vi "ref_rotary_PKP214_masterslave.vi"() -> ()   [LabVIEW 2014]
uses:
  <vilib>/eio/EIONode/EIONode.xnode
  <vilib>/rvi/FXPMathLib/FxpMul/XNode/nifxpmath_Multiplier.xnode
  <vilib>/rvi/FXPMathLib/sim/FxpSim.dll
  <vilib>/rvi/eio/common/nirviEmuTemplateMethod_errors.vi
  <vilib>/rvi/FXPMathLib/FxpSinAndCos/XNode/nifxpmath_SinAndCos.xnode
  <vilib>/rvi/FXPMathLib/FxpSinAndCos/simVIs/DllFxpSinAndCosTemp_sub.vi
  <vilib>/rvi/FXPMathLib/FxpSinAndCos/subVIs/nifxpmath_SinAndCos_SimConfig.ctl
  <vilib>/rvi/FXPMathLib/FxpSub/XNode/nifxpmath_Sub.xnode
  <vilib>/rvi/FXPMathLib/FxpAdd/XNode/nifxpmath_Add.xnode
  <vilib>/rvi/DataTransferAndStorage/Container/XNode/niFpgaContainer.xnode
  <vilib>/rvi/interface/RandomDataEmulation/nirviRandomDataFpgaMultiElementTemplate.vi
panel:
  out "omega_a (M_avg) 2":fxp<+/-,64,35>
  in  "Velocity Estimation":i16(ring) items=["M_avg method", "T method"]
  out "omega_a (M_avg)":fxp<+/-,64,35>
  in  "D_d_M_avg_Tc (uSec)":u32
  in  "theta_a_tolorence":fxp<+/-,14,3>
  in  "theta2 ratio":fxp<+/-,20,8>
  in  "tauk ratio":fxp<+/-,20,8>
  in  "tauk2_tol":fxp<+/-,20,8>
  in  "masterslave":bool
  out "Theta_ar 2":fxp<+/-,54,19>
  in  "stop motor 2":bool
  out "vb 2":fxp<+/-,38,8>
  out "va 2":fxp<+/-,38,8>
  out "vd_F 2":fxp<+/-,20,5>
  out "vq_F 2":fxp<+/-,20,5> format="%.57g"
  out "taukr_dd 2":fxp<+/-,36,29>
  out "tauk_i 2":fxp<+/-,34,18>
  in  "Kv 2":fxp<+/-,20,12>
  in  "Bv 2":fxp<+/-,20,2>
  out "taukr 2":fxp<+/-,64,31>
  out "Theta_a_error 2":fxp<+/-,24,11>
  in  "Kp 2":fxp<+/-,20,12>
  in  "Kd 2":fxp<+/-,20,8>
  out "taur 2":fxp<+/-,64,31>
  out "tauk_error 2":fxp<+/-,24,11>
  in  "Ki 2":fxp<+/-,22,9>
  in  "tauk_tolorence 2":fxp<+/-,14,3>
  out "tauk_dd 2":fxp<+/-,34,18>
  out "tauk 2":fxp<+/-,34,13>
  in  "Reduction ratio 2":fxp<+/-,20,6>
  in  "Spring stiffness 2":fxp<+/-,20,12>
  out "omega_a (rad/s)  2":fxp<+/-,32,18>
  out "omega (rad/s) 2":fxp<+/-,32,18>
  out "omega_a(T) 2":fxp<+/-,20,9>
  in  "Magnetic Encoder Reset 2":bool
  out "Magnetic Encoder Position 2":i32
  out "Theta_a 2":fxp<+/-,34,12>
  in  "Correction factor 2":fxp<+/-,24,2>
  out "mt 2":u32
  out "omega(T) 2":fxp<+/-,20,9>
  in  "Encoder Reset 2":bool
  out "Encoder Position 2":i32
  out "NrTheta 2":fxp<+/-,33,18>
  out "Thetam 2":fxp<+/-,33,18>
  in  "Correction factor":fxp<+/-,24,2>
  in  "Reduction ratio":fxp<+/-,20,6>
  out "tauk_dd":fxp<+/-,34,18>
  out "tauk":fxp<+/-,34,12>
  in  "Spring stiffness":fxp<+/-,20,12>
  in  "Kp":fxp<+/-,20,12>
  in  "Kd":fxp<+/-,20,8>
  out "taur":fxp<+/-,64,31>
  out "tauk_error":fxp<+/-,24,11>
  in  "Ki":fxp<+/-,22,9>
  in  "tauk_tolorence":fxp<+/-,14,3>
  out "omega_a (rad/s)":fxp<+/-,32,18>
  out "omega_a(T)":fxp<+/-,32,15>
  out "Theta_ar_dd":fxp<+/-,36,29>
  in  "Magnetic Encoder Reset":bool
  out "Magnetic Encoder Position":i32
  out "Theta_a":fxp<+/-,34,11>
  out "Thetam":fxp<+/-,33,18>
  out "omega(T)":fxp<+/-,32,15>
  out "Time now (s)":fxp<+,52,14>
  out "Theta_ar":fxp<+,1,1>
  out "tauk_i":fxp<+/-,34,18>
  out "Theta_a_error":fxp<+/-,24,11>
  out "taukr":fxp<+/-,64,31>
  in  "Bv":fxp<+/-,20,8>
  in  "Kv":fxp<+/-,20,12>
  out "taukr_dd":fxp<+/-,36,29>
  in  "Ini coe.":bool
  out "va":fxp<+/-,38,8>
  out "vb":fxp<+/-,38,8>
  in  "stop motor":bool
  out "vq_F":fxp<+/-,20,5> format="%.57g"
  out "vd_F":fxp<+/-,20,5>
  out "mt":u32
  out "omega (rad/s)":fxp<+/-,32,18>
  in  "mt0":u32
  out "NrTheta":fxp<+/-,33,18>
  out "Encoder Position":i32
  in  "Encoder Reset":bool
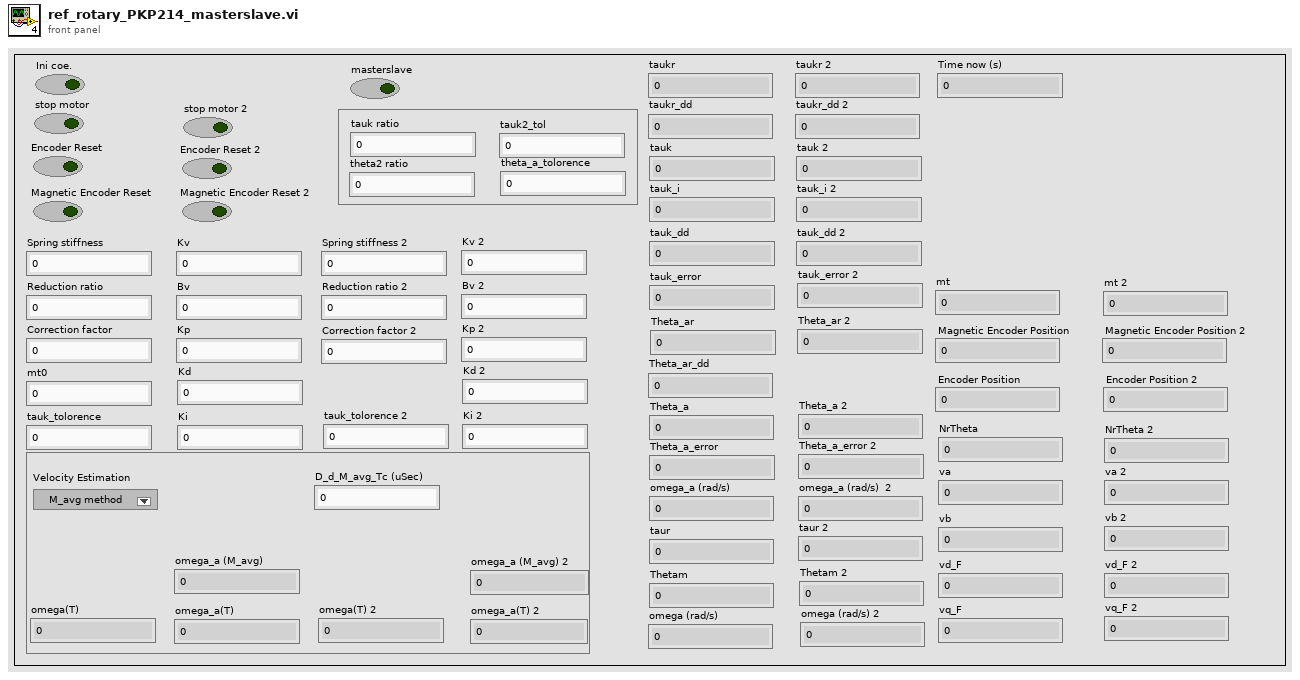
[diagram p1: front panel]
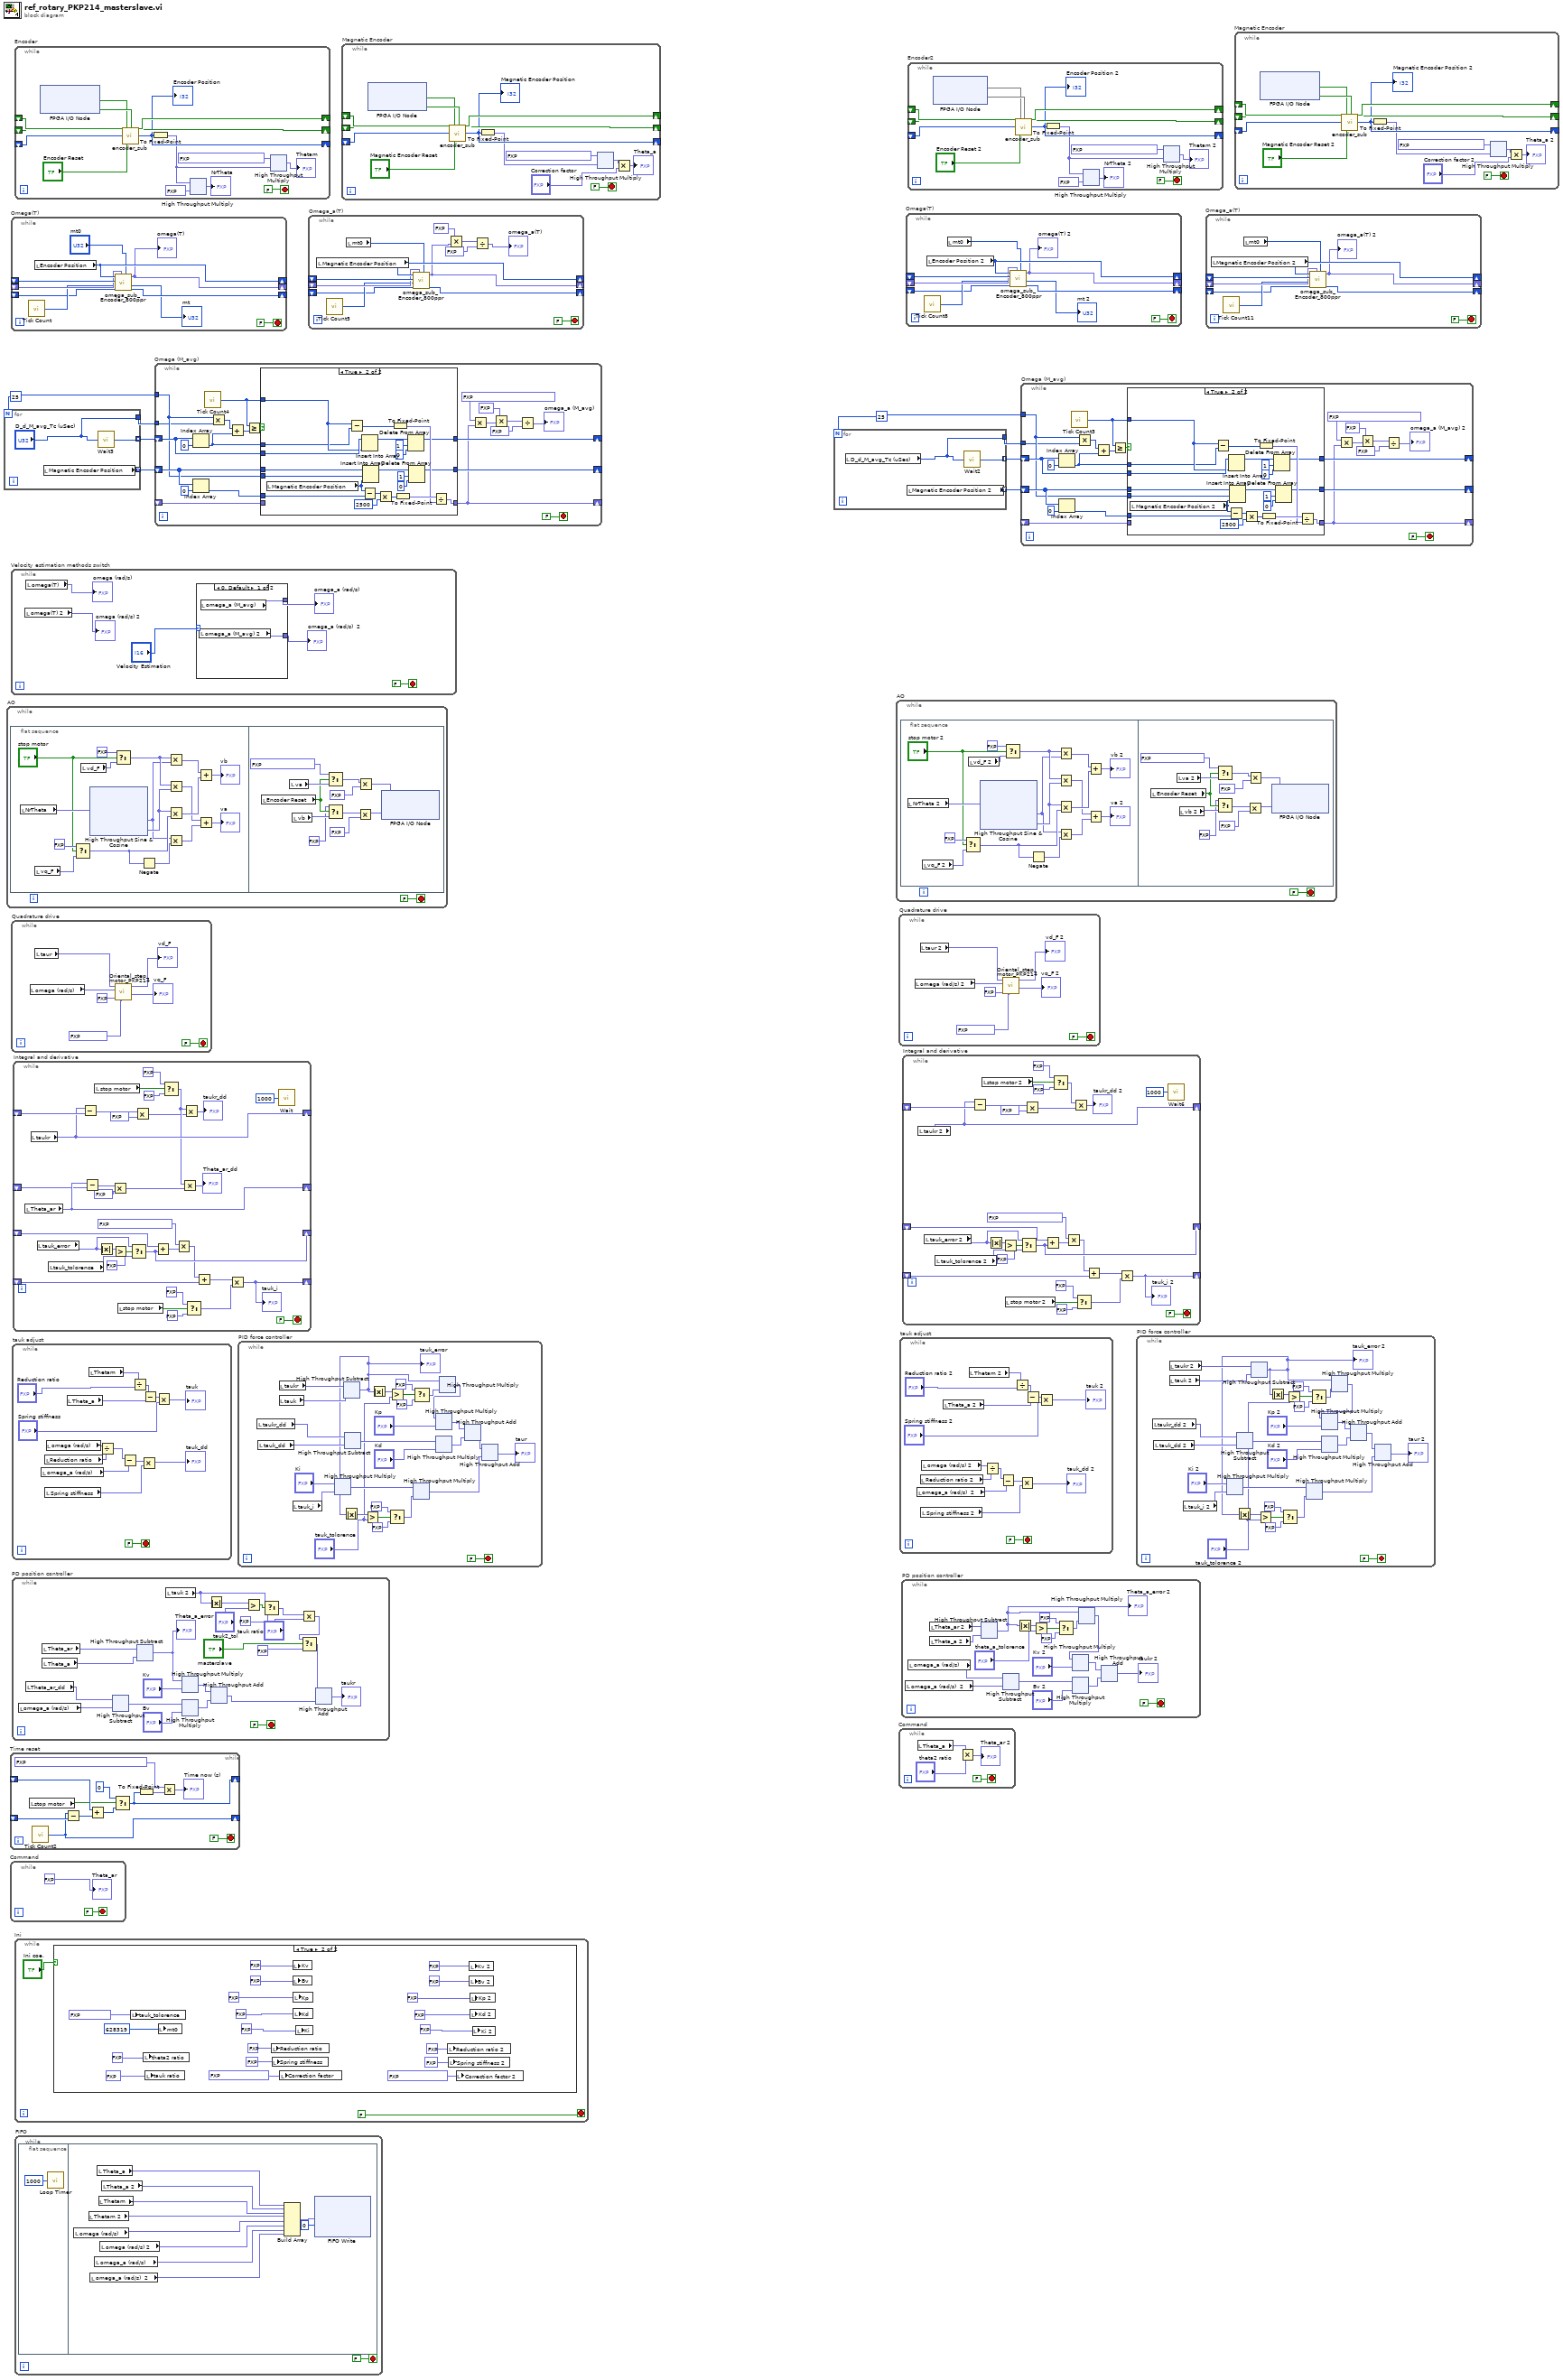
[diagram p0: block diagram]
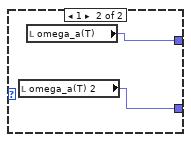
[diagram p4: hidden frame]
diagram:
  w1 = 25
  w5 = 25
  n1 = for {
    N: w5 -> [_]
    tunnel: ["D_d_M_avg_Tc (uSec)"] -> w8
    tunnel: [w11] -> w6 mode=indexing
    tunnel: [w10] -> w7 mode=indexing
    n2 = local read "Magnetic Encoder Position"() -> (w10:i32)
    n3 = call "Wait3"("Count(uSec)"="D_d_M_avg_Tc (uSec)") -> ("Tick Count(uSec)"=w11:u32)
  }
  n4 = while "AO" {
    stop <- FALSE stop-if-true
    n5 = flat-sequence {
      frame #0 {
        n6 = local read "NrTheta"() -> (w28:fxp<+/-,33,18>)
        n7 = local read "vq_F"() -> (w26:fxp<+/-,20,5>)
        n8 = Select(t=fxp<+,20,5> 0.0, s="stop motor", f=w26) -> (s? t:f=w23:fxp<+/-,21,6>)
        n9 = local read "vd_F"() -> (w27:fxp<+/-,20,5>)
        n10 = xnode "High Throughput Sine & Cosine"("x (pi)"=w28) -> ("sin(x)"=w19:fxp<+/-,17,2>, "cos(x)"=w21:fxp<+/-,17,2>)
        n11 = Select(t=fxp<+,20,5> 0.0, s="stop motor", f=w27) -> (s? t:f=w20:fxp<+/-,21,6>)
        n12 = Negate(x=w23) -> (-x=w22:fxp<+/-,21,6>)
        n13 = Multiply(x=w20, y=w19) -> (x*y=w18:fxp<+/-,37,7>)
        n14 = Multiply(x=w20, y=w21) -> (x*y=w16:fxp<+/-,37,7>)
        n15 = Multiply(x=w21, y=w23) -> (x*y=w17:fxp<+/-,37,7>)
        n16 = Multiply(x=w19, y=w22) -> (x*y=w15:fxp<+/-,37,7>)
        n17 = Add(x=w18, y=w17) -> (x+y=→"vb":fxp<+/-,38,8>)
        n18 = Add(x=w16, y=w15) -> (x+y=→"va":fxp<+/-,38,8>)
      }
      frame #1 {
        n19 = local read "Encoder Reset"() -> (w62:bool)
        n20 = local read "va"() -> (w64:fxp<+/-,38,8>)
        n21 = local read "vb"() -> (w63:fxp<+/-,38,8>)
        n22 = Select(t=fxp<+/-,20,5> 3.899993896484375 ("y"), s=w62, f=w64) -> (s? t:f=w65:fxp<+/-,38,8>)
        n23 = Select(t=fxp<+/-,20,5> 0.0 ("y"), s=w62, f=w63) -> (s? t:f=w66:fxp<+/-,38,8>)
        n24 = Multiply(x=w66, y=fxp<+/-,20,5> -0.5) -> (x*y=w70:fxp<+/-,57,12>)
        n25 = Multiply(x=w65, y=fxp<+/-,20,5> -0.5) -> (x*y=w69:fxp<+/-,57,12>)
        n26 = xnode "FPGA I/O Node"("Mod2/AO0"=w69, "Mod2/AO1"=w70) -> ()  [unwired: 2 in, 2 out]
      }
    }
  }
  n27 = while "Time reset" {
    shift-right: [w74] -> _
    shift-left: _ -> [w81]
    shift-right: [w76] -> _
    shift-left: _ -> [w77]
    stop <- FALSE stop-if-true
    n28 = local read "stop motor"() -> (w79:bool)
    n29 = call "Tick Count2"() -> ("Tick Count(uSec)"=w76:u32)
    n30 = Subtract(x=w76, y=w77) -> (x-y=w82:u32)
    n31 = Add(x=w81, y=w82) -> (x+y=w80:u32)
    n32 = Select(t=u32 0, s=w79, f=w80) -> (s? t:f=w74:u32)
    n33 = To Fixed-Point(number=w74) -> (fixed-point=w73:fxp<+,32,32>)  [unwired: 1 in]
    n34 = Multiply(x=fxp<+,20,-18> 1.0000003385357559e-06, y=w73) -> (x*y=→"Time now (s)":fxp<+,52,14>)
  }
  n35 = while "Command" {
    stop <- FALSE stop-if-true
    "Theta_ar" <- fxp<+,1,1> 0.0 ("t")
  }
  n36 = while "Omega(T)" {
    shift-right: [w93] -> _
    shift-left: _ -> [w94]
    shift-right: [w85] -> _
    shift-left: _ -> [w92]
    shift-right: [w89] -> _
    shift-left: _ -> [w90]
    stop <- FALSE stop-if-true
    n37 = call "Tick Count"() -> ("Tick Count(Ticks)"=w91:u32)
    n38 = local read "Encoder Position"() -> (w93:i32)
    n39 = call "omega_sub_Encoder_800ppr.vi"("mt0"="mt0", "omega_pre"=w92, "ticks_m_pre"=w90, "ticks"=w91, "count_pre"=w94, "count"=w93) -> ("ticks_m"=w89:u32, "mt"=→"mt":u32, "omega"=w85:fxp<+/-,20,9>)  [unwired: 3 in]
    "omega(T)" <- w85
  }
  n40 = while "Velocity estimation methods switch" {
    stop <- FALSE stop-if-true
    n41 = local read "omega(T) 2"() -> (→"omega (rad/s) 2":fxp<+/-,20,9>)
    n42 = local read "omega(T)"() -> (→"omega (rad/s)":fxp<+/-,32,15>)
    n43 = case shown="0, Default" "Velocity Estimation" {
      tunnel: [w102 w104] -> w97
      tunnel: [w101 w103] -> w96
      frame 0, Default {
        n44 = local read "omega_a (M_avg) 2"() -> (w101:fxp<+/-,64,35>)
        n45 = local read "omega_a (M_avg)"() -> (w102:fxp<+/-,64,35>)
      }
      frame 1 {
        n46 = local read "omega_a(T) 2"() -> (w103:fxp<+/-,20,9>)
        n47 = local read "omega_a(T)"() -> (w104:fxp<+/-,32,15>)
      }
    }
    "omega_a (rad/s)" <- w97
    "omega_a (rad/s)  2" <- w96
  }
  n48 = while "Quadrature drive" {
    stop <- FALSE stop-if-true
    n49 = local read "omega (rad/s)"() -> (w109:fxp<+/-,32,18>)
    n50 = local read "taur"() -> (w110:fxp<+/-,64,31>)
    n51 = call "Oriental_step_motor_PKP214.vi"("tau_Threshold"=fxp<+,16,7> 0.00390625 ("F_Threshold"), "dtaumr"=fxp<+/-,25,15> 0.0 ("dFmr"), "omega"=w109, "taumr"=w110) -> ("vq_F"=→"vq_F":fxp<+/-,20,5>, "vd_F"=→"vd_F":fxp<+/-,20,5>)  [unwired: 6 in]
  }
  n52 = while "PD position controller" {
    stop <- FALSE stop-if-true
    n53 = local read "omega_a (rad/s)"() -> (w126:fxp<+/-,32,18>)
    n54 = local read "Theta_ar_dd"() -> (w125:fxp<+/-,36,29>)
    n55 = local read "Theta_ar"() -> (w128:fxp<+,1,1>)
    n56 = local read "Theta_a"() -> (w135:fxp<+/-,34,11>)
    n57 = xnode "High Throughput Subtract"("x"=w125, "y"=w126) -> ("x-y"=w127:fxp<+/-,44,30>)
    n58 = xnode "High Throughput Subtract"("x"=w128, "y"=w135) -> ("x-y"=w129:fxp<+/-,35,12>)
    "Theta_a_error" <- w129
    n59 = local read "tauk 2"() -> (w119:fxp<+/-,34,13>)
    n60 = xnode ("High Throughput Multiply")("x"=w129, "y"="Kv") -> ("x*y"=w133:fxp<+/-,55,24>)
    n61 = xnode ("High Throughput Multiply")("x"=w127, "y"="Bv") -> ("x*y"=w132:fxp<+/-,64,38>)
    n62 = Absolute Value(x=w119) -> (abs(x)=w117:fxp<+,34,13>)
    n63 = xnode ("High Throughput Add")("x"=w133, "y"=w132) -> ("x+y"=w124:fxp<+/-,64,39>)
    n64 = Greater?(x=w117, y="tauk2_tol") -> (0:w118:bool)
    n65 = Select(t=w119, s=w118, f=fxp<+,1,1> 0.0 ("t")) -> (s? t:f=w113:fxp<+/-,34,13>)
    n66 = Multiply(x=w113, y="tauk ratio") -> (x*y=w114:fxp<+/-,54,21>)
    n67 = Select(t=w114, s="masterslave", f=fxp<+,1,1> 0.0 ("t")) -> (s? t:f=w120:fxp<+/-,54,21>)
    n68 = xnode ("High Throughput Add")("x"=w120, "y"=w124) -> ("x+y"=→"taukr":fxp<+/-,64,40>)
  }
  n69 = while "tauk adjust" {
    stop <- FALSE stop-if-true
    n70 = local read "omega_a (rad/s)"() -> (w147:fxp<+/-,32,18>)
    n71 = local read "Reduction ratio"() -> (w144:fxp<+/-,20,6>)
    n72 = local read "Spring stiffness"() -> (w145:fxp<+/-,20,12>)
    n73 = local read "omega (rad/s)"() -> (w146:fxp<+/-,32,18>)
    n74 = local read "Theta_a"() -> (w141:fxp<+/-,34,11>)
    n75 = local read "Thetam"() -> (w140:fxp<+/-,33,18>)
    n76 = Divide(x=w146, y=w144) -> (x/y=w148:fxp<+/-,53,33>)
    n77 = Subtract(x=w148, y=w147) -> (x-y=w149:fxp<+/-,53,33>)
    n78 = Divide(x=w140, y="Reduction ratio") -> (x/y=w142:fxp<+/-,54,33>)
    n79 = Multiply(x=w149, y=w145) -> (x*y=→"tauk_dd":fxp<+/-,64,44>)
    n80 = Subtract(x=w142, y=w141) -> (x-y=w143:fxp<+/-,56,33>)
    n81 = Multiply(x=w143, y="Spring stiffness") -> (x*y=→"tauk":fxp<+/-,64,44>)
  }
  n82 = while "Integral and derivative" {
    shift-right: [w181] -> _
    shift-left: _ -> [w184]
    shift-right: [w173] -> _
    shift-left: _ -> [w174]
    shift-right: [w163] -> _
    shift-left: _ -> [w167]
    shift-right: [w160] -> _
    shift-left: _ -> [w159]
    stop <- FALSE stop-if-true
    n83 = local read "Theta_ar"() -> (w160:fxp<+,1,1>)
    n84 = local read "taukr"() -> (w181:fxp<+/-,64,31>)
    n85 = local read "tauk_error"() -> (w175:fxp<+/-,24,11>)
    n86 = local read "tauk_tolorence"() -> (w178:fxp<+/-,14,3>)
    n87 = Subtract(x=w181, y=w184) -> (x-y=w183:fxp<+/-,64,32>)
    n88 = Subtract(x=w160, y=w159) -> (x-y=w162:fxp<+,1,1>)
    n89 = local read "stop motor"() -> (w156:bool)
    n90 = Absolute Value(x=w175) -> (abs(x)=w179:fxp<+,24,11>)
    n91 = Multiply(x=w162, y=fxp<+/-,33,13> 1000.0) -> (x*y=w153:fxp<+,1,-19>)
    n92 = Greater?(x=w179, y=w178) -> (0:w177:bool)
    n93 = local read "stop motor"() -> (w170:bool)
    n94 = Select(t=w175, s=w177, f=fxp<+,24,11> 0.0) -> (s? t:f=w173:fxp<+/-,25,12>)
    n95 = Multiply(x=w183, y=fxp<+/-,33,13> 1000.0) -> (x*y=w151:fxp<+/-,64,44>)
    n96 = Add(x=w174, y=w173) -> (x+y=w172:fxp<+/-,26,13>)
    n97 = Select(t=fxp<+,1,1> 0.0, s=w156, f=fxp<+,1,1> 1.0) -> (s? t:f=w152:fxp<+,1,1>)
    n98 = Multiply(x=fxp<+/-,30,12> 0.000499725341796875, y=w172) -> (x*y=w166:fxp<+/-,55,24>)
    n99 = Multiply(x=w152, y=w153) -> (x*y=→"Theta_ar_dd":fxp<+,1,-19>)
    n100 = Multiply(x=w152, y=w151) -> (x*y=→"taukr_dd":fxp<+/-,64,44>)
    n101 = Select(t=fxp<+,1,1> 0.0, s=w170, f=fxp<+,1,1> 1.0) -> (s? t:f=w164:fxp<+,1,1>)
    n102 = Add(x=w166, y=w167) -> (x+y=w165:fxp<+/-,32,16>)
    n103 = Multiply(x=w165, y=w164) -> (x*y=w163:fxp<+/-,32,16>)
    "tauk_i" <- w163
    n104 = call "Wait"("Count(uSec)"=u32 1000) -> ()  [unwired: 1 out]
  }
  n105 = while "Encoder" {
    shift-right: [w194] -> _
    shift-left: _ -> [w196]
    shift-right: [w193] -> _
    shift-left: _ -> [w195]
    shift-right: [w191] -> _
    shift-left: _ -> [w192]
    stop <- FALSE stop-if-true
    n106 = xnode "FPGA I/O Node"() -> ("Mod7/DIO2"=w199:bool, "Mod7/DIO3"=w200:bool)  [unwired: 2 in, 2 out]
    n107 = call "encoder_sub.vi"("A_pre"=w196, "B_pre"=w195, "Encoder Position_pre"=w192, "A input"=w199, "Encoder Position Reset"="Encoder Reset", "B input"=w200) -> ("A"=w194:bool, "B"=w193:bool, "Encoder Position (Counts)"=w191:i32)  [unwired: 19 in]
    "Encoder Position" <- w191
    n108 = To Fixed-Point(number=w191) -> (fixed-point=w187:fxp<+/-,32,32>)  [unwired: 1 in]
    n109 = xnode ("High Throughput Multiply")("x"=w187, "y"=fxp<+/-,24,0> 0.125) -> ("x*y"=→"NrTheta":fxp<+/-,56,32>)
    n110 = xnode ("High Throughput Multiply")("x"=fxp<+/-,24,0> 0.007853984832763672 ("y"), "y"=w187) -> ("x*y"=→"Thetam":fxp<+/-,56,32>)
  }
  n111 = while "Ini" {
    stop <- FALSE stop-if-true
    n112 = case shown="True" "Ini coe." {
      frame False {
      }
      frame True {
        n113 = local write "tauk_tolorence"(fxp<+/-,14,3> 0.009765625 ("D_tolorence")) -> ()
        n114 = local write "theta2 ratio"(fxp<+/-,16,2> 1.0 ("Dr_end")) -> ()
        n115 = local write "tauk ratio"(fxp<+/-,16,2> -0.5 ("Dr_end")) -> ()
        n116 = local write "mt0"(u32 628319 ("mt0")) -> ()
        n117 = local write "Reduction ratio"(fxp<+/-,16,11> 18.0 ("Dr_end")) -> ()
        n118 = local write "Spring stiffness"(fxp<+/-,16,11> 1.5 ("Dr_end")) -> ()
        n119 = local write "Correction factor"(fxp<+/-,16,2> 0.97235107421875 ("Dr_end")) -> ()
        n120 = local write "Kv"(fxp<+/-,16,11> 0.0 ("Dr_end")) -> ()
        n121 = local write "Bv"(fxp<+/-,16,11> 0.0 ("Dr_end")) -> ()
        n122 = local write "Kp"(fxp<+/-,20,12> 1.0 ("Kp")) -> ()
        n123 = local write "Kd"(fxp<+/-,20,8> 0.0 ("Kd")) -> ()
        n124 = local write "Ki"(fxp<+/-,24,8> 0.0 ("D_i")) -> ()
        n125 = local write "Reduction ratio 2"(fxp<+/-,16,11> 18.0 ("Dr_end")) -> ()
        n126 = local write "Spring stiffness 2"(fxp<+/-,16,11> 1.5 ("Dr_end")) -> ()
        n127 = local write "Correction factor 2"(fxp<+/-,16,2> 0.97235107421875 ("Dr_end")) -> ()
        n128 = local write "Kv 2"(fxp<+/-,16,11> 1.0 ("Dr_end")) -> ()
        n129 = local write "Bv 2"(fxp<+/-,16,11> 0.0 ("Dr_end")) -> ()
        n130 = local write "Kp 2"(fxp<+/-,20,12> 1.0 ("Kp")) -> ()
        n131 = local write "Kd 2"(fxp<+/-,20,8> 0.0 ("Kd")) -> ()
        n132 = local write "Ki 2"(fxp<+/-,24,8> 0.0 ("D_i")) -> ()
      }
    }
  }
  n133 = while "FIFO" {
    stop <- FALSE stop-if-true
    n134 = flat-sequence {
      frame #0 {
        n135 = call "Loop Timer"("Count(uSec)"=u32 1000) -> ()  [unwired: 1 out]
      }
      frame #1 {
        n136 = local read "omega (rad/s)"() -> (w225:fxp<+/-,32,18>)
        n137 = local read "Thetam 2"() -> (w229:fxp<+/-,33,18>)
        n138 = local read "omega_a (rad/s)  2"() -> (w226:fxp<+/-,32,18>)
        n139 = local read "omega_a (rad/s)"() -> (w227:fxp<+/-,32,18>)
        n140 = local read "Theta_a"() -> (w232:fxp<+/-,34,11>)
        n141 = local read "Thetam"() -> (w230:fxp<+/-,33,18>)
        n142 = local read "omega (rad/s) 2"() -> (w228:fxp<+/-,32,18>)
        n143 = local read "Theta_a 2"() -> (w231:fxp<+/-,34,12>)
        n144 = Build Array(w232, w231, w230, w229, w225, w228, w227, w226) -> (w233:fxp<+/-,41,18>[])
        n145 = xnode ("FIFO Write")("Element"=w233, "Timeout"=0) -> ()  [unwired: 1 in, 2 out]
      }
    }
  }
  n146 = while "Omega (M_avg)" {
    tunnel: w5 -> [w250]
    shift-right: [w243] -> _
    shift-left: w6 -> [w254]
    shift-right: [w242] -> _
    shift-left: _ -> [w245]
    shift-right: [w244] -> _
    shift-left: w7 -> [w253]
    tunnel: w8 -> [w247]
    stop <- FALSE stop-if-true
    n147 = Index Array(array=w254, index=0) -> (element=w248:u32)
    n148 = Index Array(array=w253, index=0) -> (element=w249:i32)
    n149 = call "Tick Count4"() -> ("Tick Count(uSec)"=w251:u32)
    n150 = Multiply(x=w250, y=w247) -> (x*y=w255:u32)
    n151 = Add(x=w255, y=w248) -> (x+y=w252:u32)
    n152 = Greater Or Equal?(x=w251, y=w252) -> (x >= y?=w246:bool)
    n153 = case shown="True" w246 {
      tunnel: w254 -> [w260 w277]
      tunnel: w253 -> [w259 w276]
      tunnel: w251 -> [_ w269]
      tunnel: w250 -> [_ w275]
      tunnel: w249 -> [_ w273]
      tunnel: w248 -> [_ w268]
      tunnel: w245 -> [w258 _]
      tunnel: [w259 w263] -> w244
      tunnel: [w260 w262] -> w243
      tunnel: [w258 w261] -> w242
      frame False {
      }
      frame True {
        n154 = local read "Magnetic Encoder Position"() -> (w274:i32)
        n155 = Subtract(x=w269, y=w268) -> (x-y=w266:u32)
        n156 = Insert Into Array(array=w277, new element=w269) -> (w278:u32[])  [unwired: 1 in]
        n157 = Subtract(x=w274, y=w273) -> (x-y=w272:i32)
        n158 = Insert Into Array(array=w276, index=w275, new element=w274) -> (w279:i32[])
        n159 = Multiply(x=w272, y=2500) -> (x*y=w270:i32)
        n160 = To Fixed-Point(number=w266) -> (fixed-point=w264:fxp<+,32,32>)  [unwired: 1 in]
        n161 = To Fixed-Point(number=w270) -> (fixed-point=w265:fxp<+/-,32,32>)  [unwired: 1 in]
        n162 = Delete From Array(array=w278, length=1, index=0) -> (array with subset deleted=w262:u32[])  [unwired: 1 out]
        n163 = Delete From Array(array=w279, length=1, index=0) -> (array with subset deleted=w263:i32[])  [unwired: 1 out]
        n164 = Divide(x=w265, y=w264) -> (x/y=w261:fxp<+/-,64,32>)
      }
    }
    n165 = Multiply(x=fxp<+/-,27,3> 3.1415926218032837, y=w242) -> (x*y=w239:fxp<+/-,64,35>)
    n166 = Multiply(x=fxp<+/-,27,14> 800.0, y=w239) -> (x*y=w237:fxp<+/-,64,49>)
    n167 = Divide(x=w237, y=fxp<+/-,27,14> 4096.0 ("x")) -> (x/y=→"omega_a (M_avg)":fxp<+/-,64,63>)
  }
  n168 = while "PID force controller" {
    stop <- FALSE stop-if-true
    n169 = local read "taukr_dd"() -> (w291:fxp<+/-,36,29>)
    n170 = local read "tauk_dd"() -> (w292:fxp<+/-,34,18>)
    n171 = local read "taukr"() -> (w294:fxp<+/-,64,31>)
    n172 = local read "tauk"() -> (w311:fxp<+/-,34,12>)
    n173 = local read "tauk_i"() -> (w304:fxp<+/-,34,18>)
    n174 = xnode ("High Throughput Multiply")("x"="Ki", "y"=w304) -> ("x*y"=w299:fxp<+/-,56,27>)
    n175 = xnode "High Throughput Subtract"("x"=w294, "y"=w311) -> ("x-y"=w285:fxp<+/-,64,32>)
    "tauk_error" <- w285
    n176 = Absolute Value(x=w285) -> (abs(x)=w303:fxp<+,64,32>)
    n177 = xnode "High Throughput Subtract"("x"=w291, "y"=w292) -> ("x-y"=w293:fxp<+/-,46,30>)
    n178 = Greater?(x=w303, y="tauk_tolorence") -> (0:w302:bool)
    n179 = Absolute Value(x=w285) -> (abs(x)=w286:fxp<+,64,32>)
    n180 = Greater?(x=w286, y="tauk_tolorence") -> (0:w288:bool)
    n181 = Select(t=fxp<+,10,2> 1.0, s=w302, f=fxp<+,10,2> 0.0) -> (s? t:f=w298:fxp<+,10,2>)
    n182 = xnode ("High Throughput Multiply")("x"=w299, "y"=w298) -> ("x*y"=w295:fxp<+/-,64,29>)
    n183 = Select(t=fxp<+,10,2> 1.0, s=w288, f=fxp<+,10,2> 0.0) -> (s? t:f=w284:fxp<+,10,2>)
    n184 = xnode ("High Throughput Multiply")("x"=w293, "y"="Kd") -> ("x*y"=w308:fxp<+/-,64,38>)
    n185 = xnode ("High Throughput Multiply")("x"=w285, "y"=w284) -> ("x*y"=w283:fxp<+/-,64,34>)
    n186 = xnode ("High Throughput Multiply")("x"=w283, "y"="Kp") -> ("x*y"=w309:fxp<+/-,64,46>)
    n187 = xnode ("High Throughput Add")("x"=w309, "y"=w308) -> ("x+y"=w296:fxp<+/-,64,47>)
    n188 = xnode ("High Throughput Add")("x"=w296, "y"=w295) -> ("x+y"=→"taur":fxp<+/-,64,48>)
  }
  n189 = while "Omega_a(T)" {
    shift-right: [w323] -> _
    shift-left: _ -> [w324]
    shift-right: [w313] -> _
    shift-left: _ -> [w322]
    shift-right: [w319] -> _
    shift-left: _ -> [w320]
    stop <- FALSE stop-if-true
    n190 = local read "Magnetic Encoder Position"() -> (w323:i32)
    n191 = call "Tick Count5"() -> ("Tick Count(Ticks)"=w321:u32)
    n192 = local read "mt0"() -> (w317:u32)
    n193 = call "omega_sub_Encoder_800ppr.vi"("mt0"=w317, "omega_pre"=w322, "ticks_m_pre"=w320, "ticks"=w321, "count_pre"=w324, "count"=w323) -> ("ticks_m"=w319:u32, "omega"=w313:fxp<+/-,20,9>)  [unwired: 3 in, 1 out]
    n194 = Multiply(x=fxp<+/-,27,14> 800.0, y=w313) -> (x*y=w316:fxp<+/-,47,23>)
    n195 = Divide(x=w316, y=fxp<+/-,27,14> 4096.0 ("x")) -> (x/y=→"omega_a(T)":fxp<+/-,64,36>)
  }
  n196 = while "Magnetic Encoder" {
    shift-right: [w334] -> _
    shift-left: _ -> [w336]
    shift-right: [w333] -> _
    shift-left: _ -> [w335]
    shift-right: [w331] -> _
    shift-left: _ -> [w332]
    stop <- FALSE stop-if-true
    n197 = xnode "FPGA I/O Node"() -> ("Mod7/DIO0"=w338:bool, "Mod7/DIO1"=w339:bool)  [unwired: 2 in, 2 out]
    n198 = call "encoder_sub.vi"("A_pre"=w336, "B_pre"=w335, "Encoder Position_pre"=w332, "A input"=w338, "Encoder Position Reset"="Magnetic Encoder Reset", "B input"=w339) -> ("A"=w334:bool, "B"=w333:bool, "Encoder Position (Counts)"=w331:i32)  [unwired: 19 in]
    "Magnetic Encoder Position" <- w331
    n199 = To Fixed-Point(number=w331) -> (fixed-point=w328:fxp<+/-,32,32>)  [unwired: 1 in]
    n200 = xnode ("High Throughput Multiply")("x"=fxp<+/-,24,0> 0.0015339851379394531 ("y"), "y"=w328) -> ("x*y"=w327:fxp<+/-,56,32>)
    n201 = Multiply(x=w327, y="Correction factor") -> (x*y=→"Theta_a":fxp<+/-,64,34>)
  }
  n202 = for {
    N: w1 -> [_]
    tunnel: [w340] -> w4
    tunnel: [w342] -> w2 mode=indexing
    tunnel: [w341] -> w3 mode=indexing
    n203 = local read "D_d_M_avg_Tc (uSec)"() -> (w340:u32)
    n204 = local read "Magnetic Encoder Position 2"() -> (w341:i32)
    n205 = call "Wait2"("Count(uSec)"=w340) -> ("Tick Count(uSec)"=w342:u32)
  }
  n206 = while "AO" {
    stop <- FALSE stop-if-true
    n207 = flat-sequence {
      frame #0 {
        n208 = local read "NrTheta 2"() -> (w359:fxp<+/-,33,18>)
        n209 = local read "vq_F 2"() -> (w357:fxp<+/-,20,5>)
        n210 = Select(t=fxp<+,20,5> 0.0, s="stop motor 2", f=w357) -> (s? t:f=w354:fxp<+/-,21,6>)
        n211 = local read "vd_F 2"() -> (w358:fxp<+/-,20,5>)
        n212 = xnode "High Throughput Sine & Cosine"("x (pi)"=w359) -> ("sin(x)"=w350:fxp<+/-,17,2>, "cos(x)"=w352:fxp<+/-,17,2>)
        n213 = Select(t=fxp<+,20,5> 0.0, s="stop motor 2", f=w358) -> (s? t:f=w351:fxp<+/-,21,6>)
        n214 = Negate(x=w354) -> (-x=w353:fxp<+/-,21,6>)
        n215 = Multiply(x=w351, y=w350) -> (x*y=w349:fxp<+/-,37,7>)
        n216 = Multiply(x=w351, y=w352) -> (x*y=w347:fxp<+/-,37,7>)
        n217 = Multiply(x=w352, y=w354) -> (x*y=w348:fxp<+/-,37,7>)
        n218 = Multiply(x=w350, y=w353) -> (x*y=w346:fxp<+/-,37,7>)
        n219 = Add(x=w349, y=w348) -> (x+y=→"vb 2":fxp<+/-,38,8>)
        n220 = Add(x=w347, y=w346) -> (x+y=→"va 2":fxp<+/-,38,8>)
      }
      frame #1 {
        n221 = local read "Encoder Reset"() -> (w393:bool)
        n222 = local read "va 2"() -> (w395:fxp<+/-,38,8>)
        n223 = local read "vb 2"() -> (w394:fxp<+/-,38,8>)
        n224 = Select(t=fxp<+/-,20,5> 3.899993896484375 ("y"), s=w393, f=w395) -> (s? t:f=w396:fxp<+/-,38,8>)
        n225 = Select(t=fxp<+/-,20,5> 0.0 ("y"), s=w393, f=w394) -> (s? t:f=w397:fxp<+/-,38,8>)
        n226 = Multiply(x=w397, y=fxp<+/-,20,5> -0.5) -> (x*y=w401:fxp<+/-,57,12>)
        n227 = Multiply(x=w396, y=fxp<+/-,20,5> -0.5) -> (x*y=w400:fxp<+/-,57,12>)
        n228 = xnode "FPGA I/O Node"("Mod2/AO2"=w400, "Mod2/AO3"=w401) -> ()  [unwired: 2 in, 2 out]
      }
    }
  }
  n229 = while "Quadrature drive" {
    stop <- FALSE stop-if-true
    n230 = local read "omega (rad/s) 2"() -> (w406:fxp<+/-,32,18>)
    n231 = local read "taur 2"() -> (w407:fxp<+/-,64,31>)
    n232 = call "Oriental_step_motor_PKP214.vi"("tau_Threshold"=fxp<+,16,7> 0.00390625 ("F_Threshold"), "dtaumr"=fxp<+/-,25,15> 0.0 ("dFmr"), "omega"=w406, "taumr"=w407) -> ("vq_F"=→"vq_F 2":fxp<+/-,20,5>, "vd_F"=→"vd_F 2":fxp<+/-,20,5>)  [unwired: 6 in]
  }
  n233 = while "Command" {
    stop <- FALSE stop-if-true
    n234 = local read "Theta_a"() -> (w411:fxp<+/-,34,11>)
    n235 = Multiply(x=w411, y="theta2 ratio") -> (x*y=→"Theta_ar 2":fxp<+/-,54,19>)
  }
  n236 = while "tauk adjust" {
    stop <- FALSE stop-if-true
    n237 = local read "omega_a (rad/s)  2"() -> (w424:fxp<+/-,32,18>)
    n238 = local read "Reduction ratio 2"() -> (w421:fxp<+/-,20,6>)
    n239 = local read "Spring stiffness 2"() -> (w422:fxp<+/-,20,12>)
    n240 = local read "omega (rad/s) 2"() -> (w423:fxp<+/-,32,18>)
    n241 = local read "Theta_a 2"() -> (w418:fxp<+/-,34,12>)
    n242 = local read "Thetam 2"() -> (w417:fxp<+/-,33,18>)
    n243 = Divide(x=w423, y=w421) -> (x/y=w425:fxp<+/-,53,33>)
    n244 = Subtract(x=w425, y=w424) -> (x-y=w426:fxp<+/-,53,33>)
    n245 = Divide(x=w417, y="Reduction ratio 2") -> (x/y=w419:fxp<+/-,54,33>)
    n246 = Multiply(x=w426, y=w422) -> (x*y=→"tauk_dd 2":fxp<+/-,64,44>)
    n247 = Subtract(x=w419, y=w418) -> (x-y=w420:fxp<+/-,55,33>)
    n248 = Multiply(x=w420, y="Spring stiffness 2") -> (x*y=→"tauk 2":fxp<+/-,64,44>)
  }
  n249 = while "PD position controller" {
    stop <- FALSE stop-if-true
    n250 = local read "omega_a (rad/s)  2"() -> (w438:fxp<+/-,32,18>)
    n251 = local read "omega_a (rad/s)"() -> (w437:fxp<+/-,32,18>)
    n252 = local read "Theta_ar 2"() -> (w440:fxp<+/-,54,19>)
    n253 = local read "Theta_a 2"() -> (w446:fxp<+/-,34,12>)
    n254 = xnode "High Throughput Subtract"("x"=w440, "y"=w446) -> ("x-y"=w431:fxp<+/-,55,20>)
    "Theta_a_error 2" <- w431
    n255 = xnode "High Throughput Subtract"("x"=w437, "y"=w438) -> ("x-y"=w439:fxp<+/-,33,19>)
    n256 = Absolute Value(x=w431) -> (abs(x)=w432:fxp<+,55,20>)
    n257 = Greater?(x=w432, y="theta_a_tolorence") -> (0:w434:bool)
    n258 = Select(t=fxp<+,10,2> 1.0, s=w434, f=fxp<+,10,2> 0.0) -> (s? t:f=w433:fxp<+,10,2>)
    n259 = xnode ("High Throughput Multiply")("x"=w439, "y"="Bv 2") -> ("x*y"=w443:fxp<+/-,53,21>)
    n260 = xnode ("High Throughput Multiply")("x"=w431, "y"=w433) -> ("x*y"=w428:fxp<+/-,64,22>)
    n261 = xnode ("High Throughput Multiply")("x"=w428, "y"="Kv 2") -> ("x*y"=w444:fxp<+/-,64,34>)
    n262 = xnode ("High Throughput Add")("x"=w444, "y"=w443) -> ("x+y"=→"taukr 2":fxp<+/-,64,35>)
  }
  n263 = while "Integral and derivative" {
    shift-right: [w471] -> _
    shift-left: _ -> [w474]
    shift-right: [w463] -> _
    shift-left: _ -> [w464]
    shift-right: [w453] -> _
    shift-left: _ -> [w457]
    stop <- FALSE stop-if-true
    n264 = local read "taukr 2"() -> (w471:fxp<+/-,64,31>)
    n265 = local read "tauk_error 2"() -> (w465:fxp<+/-,24,11>)
    n266 = local read "tauk_tolorence 2"() -> (w468:fxp<+/-,14,3>)
    n267 = Subtract(x=w471, y=w474) -> (x-y=w473:fxp<+/-,64,32>)
    n268 = local read "stop motor 2"() -> (w450:bool)
    n269 = Absolute Value(x=w465) -> (abs(x)=w469:fxp<+,24,11>)
    n270 = Greater?(x=w469, y=w468) -> (0:w467:bool)
    n271 = local read "stop motor 2"() -> (w460:bool)
    n272 = Select(t=w465, s=w467, f=fxp<+,24,11> 0.0) -> (s? t:f=w463:fxp<+/-,25,12>)
    n273 = Multiply(x=w473, y=fxp<+/-,33,13> 1000.0) -> (x*y=w447:fxp<+/-,64,44>)
    n274 = Add(x=w464, y=w463) -> (x+y=w462:fxp<+/-,26,13>)
    n275 = Select(t=fxp<+,1,1> 0.0, s=w450, f=fxp<+,1,1> 1.0) -> (s? t:f=w448:fxp<+,1,1>)
    n276 = Multiply(x=fxp<+/-,30,12> 0.000499725341796875, y=w462) -> (x*y=w456:fxp<+/-,55,24>)
    n277 = Multiply(x=w448, y=w447) -> (x*y=→"taukr_dd 2":fxp<+/-,64,44>)
    n278 = Select(t=fxp<+,1,1> 0.0, s=w460, f=fxp<+,1,1> 1.0) -> (s? t:f=w454:fxp<+,1,1>)
    n279 = Add(x=w456, y=w457) -> (x+y=w455:fxp<+/-,32,16>)
    n280 = Multiply(x=w455, y=w454) -> (x*y=w453:fxp<+/-,32,16>)
    "tauk_i 2" <- w453
    n281 = call "Wait6"("Count(uSec)"=u32 1000) -> ()  [unwired: 1 out]
  }
  n282 = while "Omega(T)" {
    shift-right: [w484] -> _
    shift-left: _ -> [w485]
    shift-right: [w477] -> _
    shift-left: _ -> [w483]
    shift-right: [w480] -> _
    shift-left: _ -> [w481]
    stop <- FALSE stop-if-true
    n283 = call "Tick Count8"() -> ("Tick Count(Ticks)"=w482:u32)
    n284 = local read "Encoder Position 2"() -> (w484:i32)
    n285 = local read "mt0"() -> (w476:u32)
    n286 = call "omega_sub_Encoder_800ppr.vi"("mt0"=w476, "omega_pre"=w483, "ticks_m_pre"=w481, "ticks"=w482, "count_pre"=w485, "count"=w484) -> ("ticks_m"=w480:u32, "mt"=→"mt 2":u32, "omega"=w477:fxp<+/-,20,9>)  [unwired: 3 in]
    "omega(T) 2" <- w477
  }
  n287 = while "Encoder2" {
    shift-right: [w494] -> _
    shift-left: _ -> [w496]
    shift-right: [w493] -> _
    shift-left: _ -> [w495]
    shift-right: [w491] -> _
    shift-left: _ -> [w492]
    stop <- FALSE stop-if-true
    n288 = xnode "FPGA I/O Node"() -> ("Mod5/DI3"=w499, "Mod5/DI4"=w500)  [unwired: 2 in, 2 out]
    n289 = call "encoder_sub.vi"("A_pre"=w496, "B_pre"=w495, "Encoder Position_pre"=w492, "A input"=w499, "Encoder Position Reset"="Encoder Reset 2", "B input"=w500) -> ("A"=w494:bool, "B"=w493:bool, "Encoder Position (Counts)"=w491:i32)  [unwired: 19 in]
    "Encoder Position 2" <- w491
    n290 = To Fixed-Point(number=w491) -> (fixed-point=w487:fxp<+/-,32,32>)  [unwired: 1 in]
    n291 = xnode ("High Throughput Multiply")("x"=w487, "y"=fxp<+/-,24,0> 0.125) -> ("x*y"=→"NrTheta 2":fxp<+/-,56,32>)
    n292 = xnode ("High Throughput Multiply")("x"=fxp<+/-,24,0> 0.007853984832763672 ("y"), "y"=w487) -> ("x*y"=→"Thetam 2":fxp<+/-,56,32>)
  }
  n293 = while "Omega (M_avg)" {
    tunnel: w1 -> [w516]
    shift-right: [w509] -> _
    shift-left: w2 -> [w520]
    shift-right: [w508] -> _
    shift-left: _ -> [w511]
    shift-right: [w510] -> _
    shift-left: w3 -> [w519]
    tunnel: w4 -> [w513]
    stop <- FALSE stop-if-true
    n294 = Index Array(array=w520, index=0) -> (element=w514:u32)
    n295 = Index Array(array=w519, index=0) -> (element=w515:i32)
    n296 = call "Tick Count3"() -> ("Tick Count(uSec)"=w517:u32)
    n297 = Multiply(x=w516, y=w513) -> (x*y=w521:u32)
    n298 = Add(x=w521, y=w514) -> (x+y=w518:u32)
    n299 = Greater Or Equal?(x=w517, y=w518) -> (x >= y?=w512:bool)
    n300 = case shown="True" w512 {
      tunnel: w520 -> [w526 w543]
      tunnel: w519 -> [w525 w542]
      tunnel: w517 -> [_ w535]
      tunnel: w516 -> [_ w541]
      tunnel: w515 -> [_ w539]
      tunnel: w514 -> [_ w534]
      tunnel: w511 -> [w524 _]
      tunnel: [w525 w529] -> w510
      tunnel: [w526 w528] -> w509
      tunnel: [w524 w527] -> w508
      frame False {
      }
      frame True {
        n301 = local read "Magnetic Encoder Position 2"() -> (w540:i32)
        n302 = Subtract(x=w535, y=w534) -> (x-y=w532:u32)
        n303 = Insert Into Array(array=w543, new element=w535) -> (w544:u32[])  [unwired: 1 in]
        n304 = Subtract(x=w540, y=w539) -> (x-y=w538:i32)
        n305 = Insert Into Array(array=w542, index=w541, new element=w540) -> (w545:i32[])
        n306 = Multiply(x=w538, y=2500) -> (x*y=w536:i32)
        n307 = To Fixed-Point(number=w532) -> (fixed-point=w530:fxp<+,32,32>)  [unwired: 1 in]
        n308 = To Fixed-Point(number=w536) -> (fixed-point=w531:fxp<+/-,32,32>)  [unwired: 1 in]
        n309 = Delete From Array(array=w544, length=1, index=0) -> (array with subset deleted=w528:u32[])  [unwired: 1 out]
        n310 = Delete From Array(array=w545, length=1, index=0) -> (array with subset deleted=w529:i32[])  [unwired: 1 out]
        n311 = Divide(x=w531, y=w530) -> (x/y=w527:fxp<+/-,64,32>)
      }
    }
    n312 = Multiply(x=fxp<+/-,27,3> 3.1415926218032837, y=w508) -> (x*y=w505:fxp<+/-,64,35>)
    n313 = Multiply(x=fxp<+/-,27,14> 800.0, y=w505) -> (x*y=w503:fxp<+/-,64,49>)
    n314 = Divide(x=w503, y=fxp<+/-,27,14> 4096.0 ("x")) -> (x/y=→"omega_a (M_avg) 2":fxp<+/-,64,63>)
  }
  n315 = while "PID force controller" {
    stop <- FALSE stop-if-true
    n316 = local read "taukr_dd 2"() -> (w557:fxp<+/-,36,29>)
    n317 = local read "tauk_dd 2"() -> (w558:fxp<+/-,34,18>)
    n318 = local read "taukr 2"() -> (w560:fxp<+/-,64,31>)
    n319 = local read "tauk 2"() -> (w577:fxp<+/-,34,13>)
    n320 = local read "tauk_i 2"() -> (w570:fxp<+/-,34,18>)
    n321 = xnode ("High Throughput Multiply")("x"="Ki 2", "y"=w570) -> ("x*y"=w565:fxp<+/-,56,27>)
    n322 = xnode "High Throughput Subtract"("x"=w557, "y"=w558) -> ("x-y"=w559:fxp<+/-,46,30>)
    n323 = xnode "High Throughput Subtract"("x"=w560, "y"=w577) -> ("x-y"=w552:fxp<+/-,64,32>)
    "tauk_error 2" <- w552
    n324 = Absolute Value(x=w552) -> (abs(x)=w569:fxp<+,64,32>)
    n325 = Greater?(x=w569, y="tauk_tolorence 2") -> (0:w568:bool)
    n326 = Absolute Value(x=w552) -> (abs(x)=w551:fxp<+,64,32>)
    n327 = Select(t=fxp<+,10,2> 1.0, s=w568, f=fxp<+,10,2> 0.0) -> (s? t:f=w564:fxp<+,10,2>)
    n328 = Greater?(x=w551, y="tauk_tolorence 2") -> (0:w554:bool)
    n329 = xnode ("High Throughput Multiply")("x"=w565, "y"=w564) -> ("x*y"=w561:fxp<+/-,64,29>)
    n330 = Select(t=fxp<+,10,2> 1.0, s=w554, f=fxp<+,10,2> 0.0) -> (s? t:f=w553:fxp<+,10,2>)
    n331 = xnode ("High Throughput Multiply")("x"=w559, "y"="Kd 2") -> ("x*y"=w574:fxp<+/-,64,38>)
    n332 = xnode ("High Throughput Multiply")("x"=w552, "y"=w553) -> ("x*y"=w549:fxp<+/-,64,34>)
    n333 = xnode ("High Throughput Multiply")("x"=w549, "y"="Kp 2") -> ("x*y"=w575:fxp<+/-,64,46>)
    n334 = xnode ("High Throughput Add")("x"=w575, "y"=w574) -> ("x+y"=w562:fxp<+/-,64,47>)
    n335 = xnode ("High Throughput Add")("x"=w562, "y"=w561) -> ("x+y"=→"taur 2":fxp<+/-,64,48>)
  }
  n336 = while "Omega_a(T)" {
    shift-right: [w585] -> _
    shift-left: _ -> [w586]
    shift-right: [w579] -> _
    shift-left: _ -> [w584]
    shift-right: [w581] -> _
    shift-left: _ -> [w582]
    stop <- FALSE stop-if-true
    n337 = local read "Magnetic Encoder Position 2"() -> (w585:i32)
    n338 = call "Tick Count11"() -> ("Tick Count(Ticks)"=w583:u32)
    n339 = local read "mt0"() -> (w578:u32)
    n340 = call "omega_sub_Encoder_800ppr.vi"("mt0"=w578, "omega_pre"=w584, "ticks_m_pre"=w582, "ticks"=w583, "count_pre"=w586, "count"=w585) -> ("ticks_m"=w581:u32, "omega"=w579:fxp<+/-,20,9>)  [unwired: 3 in, 1 out]
    "omega_a(T) 2" <- w579
  }
  n341 = while "Magnetic Encoder" {
    shift-right: [w596] -> _
    shift-left: _ -> [w598]
    shift-right: [w595] -> _
    shift-left: _ -> [w597]
    shift-right: [w593] -> _
    shift-left: _ -> [w594]
    stop <- FALSE stop-if-true
    n342 = xnode "FPGA I/O Node"() -> ("Mod7/DIO4"=w600:bool, "Mod7/DIO5"=w601:bool)  [unwired: 2 in, 2 out]
    n343 = call "encoder_sub.vi"("A_pre"=w598, "B_pre"=w597, "Encoder Position_pre"=w594, "A input"=w600, "Encoder Position Reset"="Magnetic Encoder Reset 2", "B input"=w601) -> ("A"=w596:bool, "B"=w595:bool, "Encoder Position (Counts)"=w593:i32)  [unwired: 19 in]
    "Magnetic Encoder Position 2" <- w593
    n344 = To Fixed-Point(number=w593) -> (fixed-point=w590:fxp<+/-,32,32>)  [unwired: 1 in]
    n345 = xnode ("High Throughput Multiply")("x"=fxp<+/-,24,0> 0.0015339851379394531 ("y"), "y"=w590) -> ("x*y"=w589:fxp<+/-,56,32>)
    n346 = Multiply(x=w589, y="Correction factor 2") -> (x*y=→"Theta_a 2":fxp<+/-,64,34>)
  }
